vi "pass fail action decision.vi"(6 "Communication Type":T1, 7 "fail behavior":T3, 8 "Motion":T2, 9 "Pass?":bool, 10 "Sequence State in":T4, 11 "event queue in":string[](array[string])) -> (2 "Sequence State out":T4, 3 "Event queue out":string[](array[string]))   [LabVIEW 2018]
uses:
  02.Type Def's/sequence state.ctl
  05.UserVI's/sequence/type defs/Sequence Info.ctl
  02.Type Def's/failure behaviors.ctl
  02.Type Def's/All Motions.ctl
  02.Type Def's/All Communication Types.ctl
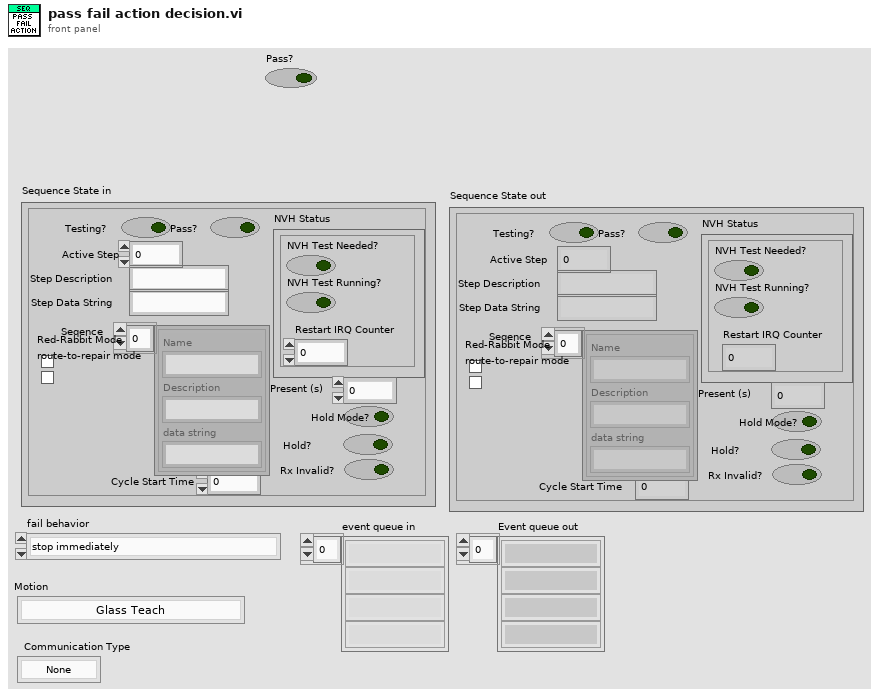
[diagram p1: front panel]
types:
  T1 = typedef "All Communication Types.ctl" = enum16{"None", "CAN", "RS 232", "RS 232 LIN", "GM LIN", "SnT LIN", "K Line", "Robel CAN", "P42M-Continental", "Inalfa SCU LIN", "Spare 3"}
  T2 = typedef "All Motions.ctl" = enum16{"Glass Teach", "Glass Slide Open", "Glass Slide Close", "Glass Vent Open", "Glass Vent Close", "Sunshade Teach", "Sunshade Open", "Sunshade Close", "Idle", "Sunshade Open 2", "Sunshade Close 2", "Glass Slide Open Sunshade Open", "Glass Slide Open Sunshade Close", "Glass Slide Close Sunshade Open", "Glass Slide Close Sunshade Close", "Glass Vent Open Sunshade Open", "Glass Vent Open Sunshade Close", "Glass Vent Close Sunshade Open", "Glass Vent Close Sunshade Close", "Express Glass Slide Open", "Express Glass Slide Close", "Express Glass Vent Open", "Express Glass Vent Close", "Express Sunshade Open", "Express Sunshade Close", "Express Sunshade Open 2", "Express Sunshade Close 2", "Express Glass Slide Open Sunshade Open", "Express Glass Slide Open Sunshade Close", "Express Glass Slide Close Sunshade Open", "Express Glass Slide Close Sunshade Close", "Express Glass Vent Open Sunshade Open", "Express Glass Vent Open Sunshade Close", "Express Glass Vent Close Sunshade Open", "Express Glass Vent Close Sunshade Close", "Goto Position Glass", "Goto Position Sunshade", "Sunshade Teach 2"}
  T3 = typedef "failure behaviors.ctl" = enum16{"stop immediately", "stop immediately if not rabbit", "stop at next 'check sequence' if not rabbit"}
  T4 = typedef "sequence state.ctl" = cluster{"Step Description":string, "Cycle Start Time":u32, "Step Data String":string, "Pass?":bool, "Seqence":T5[], "Active Step":u8, "Testing?":bool, "Red-Rabbit Mode":bool, "route-to-repair mode":bool, "NVH Status":cluster{"Restart IRQ Counter":u8, "NVH Test Needed?":bool, "NVH Test Running?":bool}, "Present (s)":dbl, "Hold Mode?":bool, "Hold?":bool, "Rx Invalid?":bool}
  T5 = typedef "Sequence Info.ctl" = cluster{"Name":string, "Description":string, "data string":string}
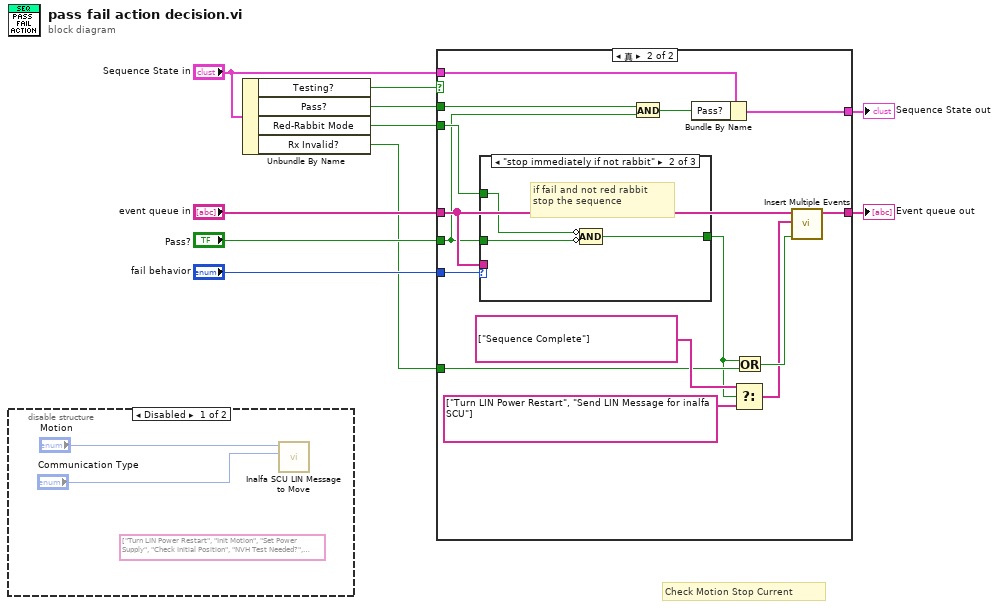
[diagram p0: block diagram]
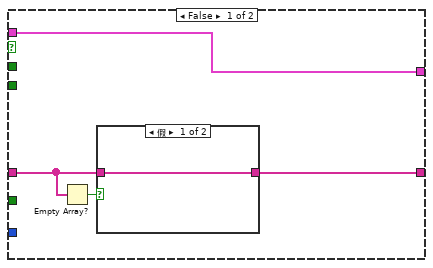
[diagram p3: hidden frame]
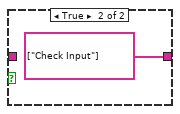
[diagram p4: hidden frame]
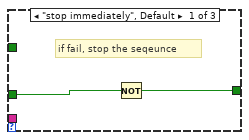
[diagram p5: hidden frame]
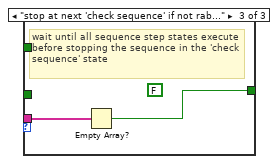
[diagram p6: hidden frame]
diagram:
  # "Check Motion Stop Current"
  n1 = disable-structure shown="Disabled" {
    frame Disabled {
      (unwired) string[] ["Turn LIN Power Restart", "Init Motion", "Set Power Supply", "Check Initial Position", "NVH Test Needed?", "Check Enter AP Message Mode", "Send LIN Message for inalfa SCU", "Check Switch Signals", "Check Initial Motion", "Get Data"] ("event queue out")
      n2 = call "Inalfa SCU LIN Message to Move.vi"("Communication Type"="Communication Type", "Motion"="Motion") -> ()  [unwired: 9 in, 1 out]
    }
    frame Enabled {
    }
  }
  n3 = Unbundle By Name("Sequence State in") -> ("Testing?"=w2:bool, "Pass?"=w10:bool, "Red-Rabbit Mode"=w4:bool, "Rx Invalid?"=w1:bool)
  n4 = case shown="真" w2 {
    tunnel: w10 -> [_ w33]
    tunnel: [w16 w31] -> w9
    tunnel: "Sequence State in" -> [w16 w30]
    tunnel: [w14 w29] -> w7
    tunnel: "event queue in" -> [w13 w26]
    tunnel: "fail behavior" -> [_ w28]
    tunnel: w4 -> [_ w27]
    tunnel: "Pass?" -> [_ w22]
    tunnel: w1 -> [_ w21]
    frame False {
      n5 = Empty Array?(array=w13) -> (empty?=w15:bool)
      n6 = case shown="假" w15 {
        tunnel: [w17 string[] ["Check Input"] ("event queue in")] -> w14
        tunnel: w13 -> [w17 _]
        frame False {
        }
        frame True {
        }
      }
    }
    frame True {
      n7 = case shown="\"stop immediately if not rabbit\"" w28 {
        tunnel: w27 -> [_ w37 _]
        tunnel: w22 -> [w35 w38 _]
        tunnel: [w34 w36 w39] -> w19
        tunnel: w26 -> [_ _ w40]
        frame "stop immediately", Default {
          # "if fail, stop the seqeunce"
          n8 = Not(x=w35) -> (.not. x?=w34:bool)
        }
        frame "stop immediately if not rabbit" {
          # "if fail and not red rabbit\nstop the sequence"
          n9 = Compound Arithmetic op=AND(invert w37, invert w38) -> (w36:bool)
        }
        frame "stop at next 'check sequence' if not rabbit" {
          (unwired) FALSE
          # "wait until all sequence step states execute before stopping the sequence in the 'check sequence' state"
          n10 = Empty Array?(array=w40) -> (empty?=w39:bool)
        }
      }
      n11 = And(x=w33, y=w22) -> (x .and. y?=w32:bool)
      n12 = Bundle By Name(cluster=w30, "Pass?"=w32) -> (w31:T4)
      n13 = Select(t=string[] ["Sequence Complete"] ("Events to Insert"), s=w19, f=string[] ["Turn LIN Power Restart", "Send LIN Message for inalfa SCU"] ("Events to Insert")) -> (s? t:f=w23:string[])
      n14 = Or(x=w19, y=w21) -> (x .or. y?=w24:bool)
      n15 = call "Insert Multiple Events.vi"("Insert all? (T)"=w24, "Events to Insert"=w23, "Event queue in"=w26) -> ("Event queue out"=w29:string[])  [unwired: 4 in]
    }
  }
  "Sequence State out" <- w9
  "Event queue out" <- w7
